vi "Navigation.vi"(8 "error in":errorcluster, 10 "Array of path nodes":T1, 11 "Robot current position":T2) -> (0 "error out":errorcluster, 3 "Movements":cluster{"Left":dbl, "Right":dbl}[](array[cluster]))   [LabVIEW 2009, in "Main.lvlib"]
doc: "Main navigation algorithm. Takes the planned path and outputs corresponding relative movements to the drive algorithm."
uses:
  Main.lvlib
  Navigation/Nav_CordinateArray.ctl
  Drive/Drive_PositionControlMode.ctl
  Navigation.lvlib
  Drive.lvlib
panel:
  in  "Travel Short Distance":bool=TRUE
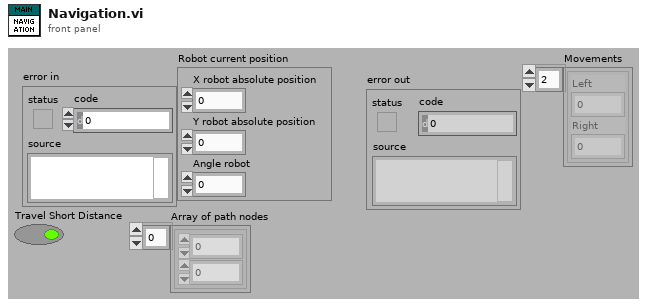
[diagram p1: front panel]
types:
  T1 = typedef "Navigation.lvlib/Nav_CordinateArray.ctl" = cluster{"X position":dbl, "Y position":dbl}[]
  T2 = cluster{"X robot absolute position":dbl, "Y robot absolute position":dbl, "Angle robot":dbl}
  T3 = typedef "Drive.lvlib/Drive_PositionControlMode.ctl" = enum16{"TurnThenStraight"}
  T4 = typedef "Navigation.lvlib/Nav_Cordinates.ctl" = cluster{"X position":dbl, "Y position":dbl}
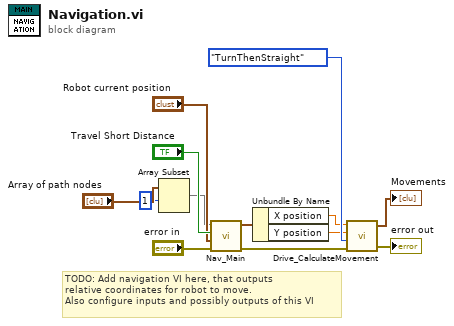
[diagram p0: block diagram]
diagram:
  # "TODO: Add navigation VI here, that outputs\nrelative coordinates for robot to move.\nAlso configure inputs and possibly outputs of this VI"
  n1 = Array Subset(array="Array of path nodes", index=1) -> (w2:T1)  [unwired: 1 in]
  n2 = call "Nav_Main.vi"("error in"="error in", "Robot current position"="Robot current position", "Travel Short Distance"="Travel Short Distance", "Array of path nodes"=w2) -> ("error out"=w11:errorcluster, "Output X and Y"=w9:T4)  [unwired: 6 in]
  n3 = Unbundle By Name(w9) -> ("X position"=w8:dbl, "Y position"=w7:dbl)
  n4 = call "Drive_CalculateMovement.vi"("error in"=w11, "Mode"=Drive_PositionControlMode."TurnThenStraight", "Y rel"=w7, "X rel"=w8) -> ("error out"=→"error out":errorcluster, "Movements"=→"Movements":cluster{"Left":dbl, "Right":dbl}[])  [unwired: 1 in]
